vi "Race.vi"() -> ()   [LabVIEW 2015]
panel:
  out "Numeric":dbl
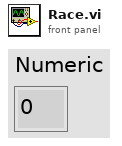
[diagram p1: front panel]
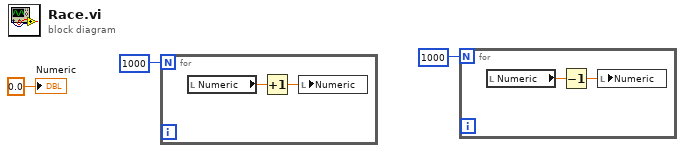
[diagram p0: block diagram]
diagram:
  n1 = for {
    N: 1000 -> [_]
    n2 = local read "Numeric"() -> (w5:dbl)
    n3 = Increment(x=w5) -> (x+1=w4:dbl)
    n4 = local write "Numeric"(w4) -> ()
  }
  n5 = for {
    N: 1000 -> [_]
    n6 = local read "Numeric"() -> (w7:dbl)
    n7 = Decrement(x=w7) -> (x-1=w6:dbl)
    n8 = local write "Numeric"(w6) -> ()
  }
  "Numeric" <- 0.0 ("Numeric")
